vi "Pressure Setpoint.vi"(7 "Set? (F:Read)":bool, 8 "Error In":errorcluster, 9 "Pressure Setpoint (0%)":dbl, 11 "VISA resource name":refnum<visa-resource-name>) -> (0 "Error Out":errorcluster, 1 "Pressure Setpoint out":dbl, 3 "dup VISA resource name":refnum<visa-resource-name>)   [LabVIEW 2011, in "MGC647C.lvlib"]
doc: "Enter pressure setpoint."
uses:
  <instrlib>/MGC647C/MGC647C.lvlib
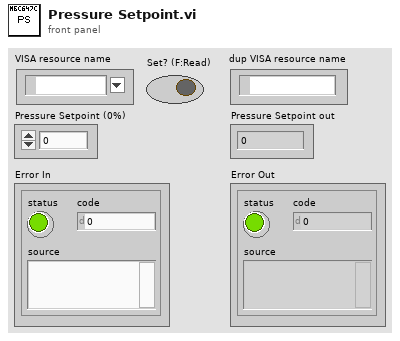
[diagram p1: front panel]
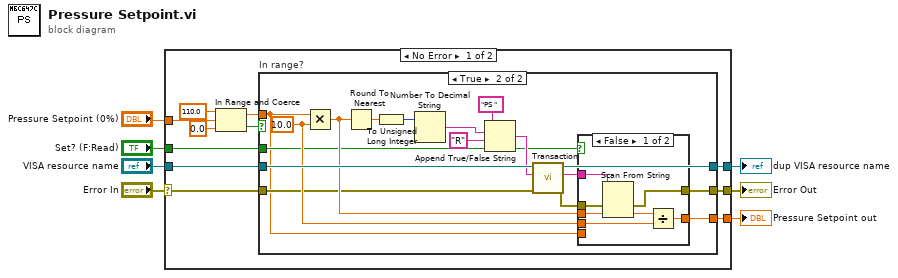
[diagram p0: block diagram]
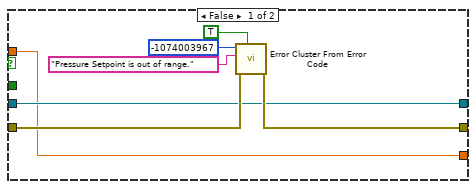
[diagram p2: hidden frame]
diagram:
  n1 = case shown="No Error" "Error In" {
    selector: "Error In" -> [w10 w53]
    tunnel: "VISA resource name" -> [w18 w52]
    tunnel: [w17 w52] -> w6
    tunnel: [w16 w53] -> w5
    tunnel: "Set? (F:Read)" -> [w15 _]
    tunnel: "Pressure Setpoint (0%)" -> [w14 w54]
    tunnel: [w9 w54] -> w1
    frame No Error {
      n2 = In Range and Coerce(upper limit=110.0, x=w14, lower limit=0.0) -> (coerced(x)=w13:dbl, In Range?=w8:bool)
      n3 = case "In range?" shown="True" w8 {
        tunnel: w18 -> [w23 w42]
        tunnel: [w23 w41] -> w17
        tunnel: [w24 w38] -> w16
        tunnel: w15 -> [_ w27]
        tunnel: w13 -> [w22 w26]
        tunnel: w10 -> [w25 w30]
        tunnel: [w22 w36] -> w9
        frame False {
          n4 = call <vilib>:"Error Cluster From Error Code.vi"("show call chain? (False)"=TRUE, "error in (no error)"=w25, "error message (\"\")"="Pressure Setpoint is out of range." ("error message (\"\")"), "error code (0)"=-1074003967) -> ("error out"=w24:errorcluster)  [unwired: 5 in]
        }
        frame True {
          w35 = 10.0 ("y")
          n5 = Multiply(x=w26, y=w35) -> (x*y=w34:dbl)
          n6 = Round To Nearest(number=w34) -> (nearest integer value=w37:dbl)
          n7 = To Unsigned Long Integer(number=w37) -> (unsigned 32bit integer=w29:u32)
          n8 = Number To Decimal String(number=w29) -> (decimal integer string=w28:string)  [unwired: 1 in]
          n9 = Append True/False String(1:w27, 2:"R" ("false string"), 3:w28, 4:"PS " ("string (\"\")")) -> (0:w32:string)
          n10 = call <instrlib>:"Transaction.vi"("Error In"=w30, "Command"=w32, "VISA resource name"=w42) -> ("Error Out"=w39:errorcluster, "Response"=w40:string, "dup VISA resource name"=w41:refnum<visa-resource-name>)  [unwired: 6 in]
          n11 = case shown="False" w27 {
            tunnel: w40 -> [w49 _]
            tunnel: w39 -> [w48 w51]
            tunnel: [w47 w51] -> w38
            tunnel: [w45 w50] -> w36
            tunnel: w35 -> [w44 _]
            tunnel: w34 -> [w43 _]
            tunnel: w26 -> [_ w50]
            frame False {
              n12 = Scan From String(input string=w49, error in=w48, default 1=w43) -> (error out=w47:errorcluster, output 1=w46:dbl)  [unwired: 2 in, 2 out]
              n13 = Divide(x=w46, y=w44) -> (x/y=w45:dbl)
            }
            frame True {
            }
          }
        }
      }
    }
    frame Error {
    }
  }
  "dup VISA resource name" <- w6
  "Error Out" <- w5
  "Pressure Setpoint out" <- w1
